vi "Configure Scaling.vi"(5 "sigma value":dbl=0.0001 min=0.0001 max=99999.9999 step=1e-07, 7 "status":bool, 8 "error in":errorcluster, 9 "channel status":u16(ring) items=["VT", "CT", "SFAC", "STAT"], 10 "channel":i32(ring) items=["All", "ELEM1", "ELEM2", "ELEM3", "ELEM4", "ELEM5", "ELEM6", "ELEM7", "SIGMA", "SIGMB", "SIGMC"], 11 "VISA resource name":refnum<visa-resource-name>) -> (0 "error out":errorcluster, 3 "VISA resource out":refnum<visa-resource-name>)   [LabVIEW 2018, in "Suita SPAW7000.lvlib"]
uses:
  <instrlib>/Suita SPAW7000/Suita SPAW7000.lvlib
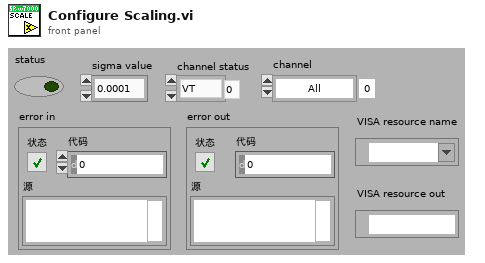
[diagram p1: front panel]
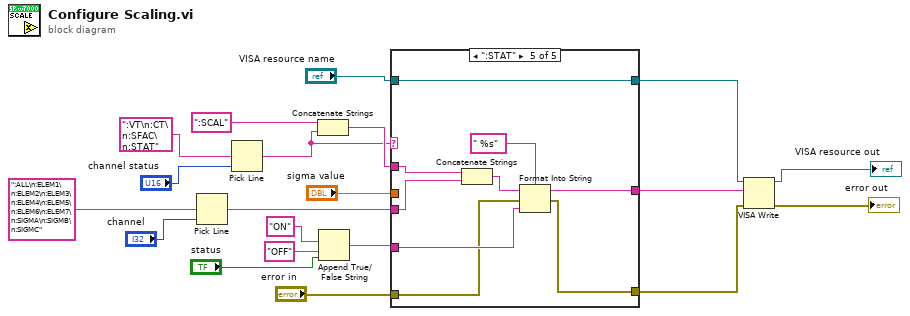
[diagram p0: block diagram]
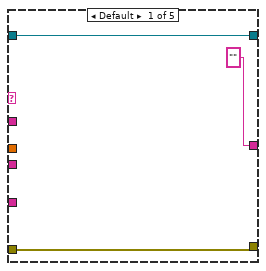
[diagram p2: hidden frame]
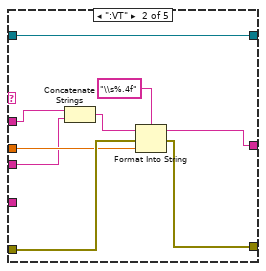
[diagram p3: hidden frame]
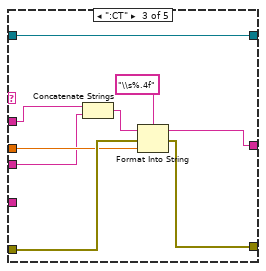
[diagram p4: hidden frame]
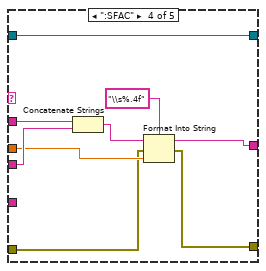
[diagram p5: hidden frame]
diagram:
  n1 = Pick Line(multi-line string=":ALL\n:ELEM1\n:ELEM2\n:ELEM3\n:ELEM4\n:ELEM5\n:ELEM6\n:ELEM7\n:SIGMA\n:SIGMB\n:SIGMC", line index="channel") -> (output string=w15:string)  [unwired: 1 in]
  n2 = Pick Line(multi-line string=":VT\n:CT\n:SFAC\n:STAT", line index="channel status") -> (output string=w12:string)  [unwired: 1 in]
  n3 = Concatenate Strings(":SCAL", w12) -> (w13:string)
  n4 = Append True/False String(1:"status", 2:"OFF" ("假字符串"), 3:"ON" ("真字符串")) -> (0:w1:string)  [unwired: 1 in]
  n5 = case shown="\":STAT\"" w12 {
    tunnel: w15 -> [_ w24 w35 w48 w55]
    tunnel: "error in" -> [w22 w29 w38 w45 w52]
    tunnel: [w22 w26 w34 w44 w51] -> w9
    tunnel: "VISA resource name" -> [w23 w32 w41 w50 w59]
    tunnel: [w23 w32 w41 w50 w59] -> w6
    tunnel: ["" w25 w33 w42 w57] -> w5
    tunnel: w13 -> [_ w27 w36 w49 w56]
    tunnel: w1 -> [_ _ _ _ w58]
    tunnel: "sigma value" -> [_ w28 w37 w46 _]
    frame Default {
    }
    frame ":VT" {
      n6 = Concatenate Strings(w27, w24) -> (w31:string)
      n7 = Format Into String(format string="\\s%.4f" ("格式字符串"), initial string=w31, error in=w29, w28) -> (resulting string=w25:string, error out=w26:errorcluster)
    }
    frame ":CT" {
      n8 = Concatenate Strings(w36, w35) -> (w40:string)
      n9 = Format Into String(format string="\\s%.4f" ("格式字符串"), initial string=w40, error in=w38, w37) -> (resulting string=w33:string, error out=w34:errorcluster)
    }
    frame ":SFAC" {
      n10 = Concatenate Strings(w49, w48) -> (w47:string)
      n11 = Format Into String(format string="\\s%.4f" ("格式字符串"), initial string=w47, error in=w45, w46) -> (resulting string=w42:string, error out=w44:errorcluster)
    }
    frame ":STAT" {
      n12 = Concatenate Strings(w56, w55) -> (w54:string)
      n13 = Format Into String(format string=" %s" ("格式字符串"), initial string=w54, error in=w52, w58) -> (resulting string=w57:string, error out=w51:errorcluster)
    }
  }
  n14 = VISA Write(VISA resource name=w6, write buffer=w5, error in (no error)=w9) -> (VISA resource name out=→"VISA resource out":refnum<visa-resource-name>, error out=→"error out":errorcluster)  [unwired: 1 out]
